vi "Generation Mode.vi"(8 "error in (no error)":errorcluster, 10 "Generation Mode":T1, 11 "PXIe5413 in":refnum<class "PXIe5413.lvclass">) -> (0 "error out":errorcluster, 3 "PXIe5413 out":refnum<class "PXIe5413.lvclass">)   [LabVIEW 2018, in "PXIe5413.lvlib" / "PXIe5413.lvclass"]
uses:
  PXIe5413.lvclass
  PPLs/Function Generator/Parent/Function Generator.lvlibp/Custom Controls/Generation Mode.ctl
  PPLs/Function Generator/Parent/Function Generator.lvlibp/Function Generator.lvclass
  C:/Projects/LabVIEW/PPLs/Function Generator/Parent/Function Generator.lvlibp/Function Generator.lvclass
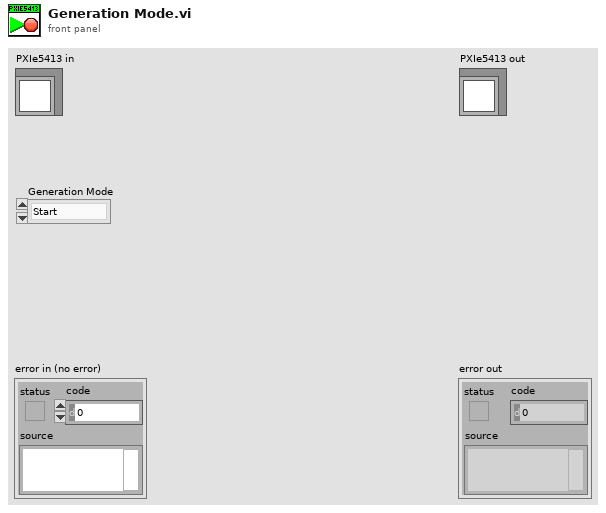
[diagram p1: front panel]
types:
  T1 = typedef "Function Generator.lvlibp/Function Generator.lvclass/Generation Mode.ctl" = enum16{"Start", "Stop"}
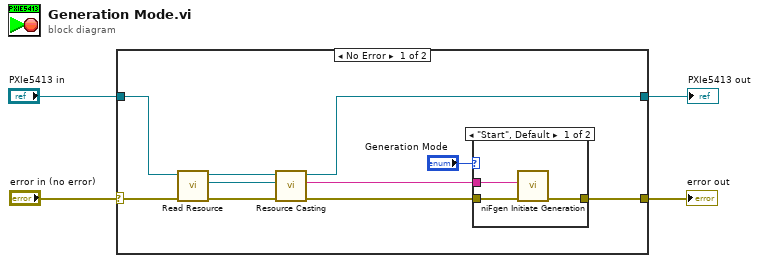
[diagram p0: block diagram]
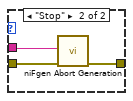
[diagram p2: hidden frame]
diagram:
  n1 = case shown="No Error" "error in (no error)" {
    selector: "error in (no error)" -> [w13 w22]
    tunnel: [w7 w22] -> w3
    tunnel: [w6 w21] -> w2
    tunnel: "PXIe5413 in" -> [w14 w21]
    frame No Error {
      n2 = call "Read Resource.vi"("error in (no error)"=w13, "Function Generator in"=w14) -> ("error out"=w12:errorcluster, "Resource"=w5:refnum<visa-resource-name>, "Function Generator out"=w11:refnum<class "PXIe5413.lvclass">)  [unwired: 7 in]
      n3 = call "Resource Casting.vi"("error in (no error)"=w12, "VISA Resource In"=w5, "PXIe5413 in"=w11) -> ("error out"=w10:errorcluster, "Casted Resource"=w8:string, "PXIe5413 out"=w6:refnum<class "PXIe5413.lvclass">)  [unwired: 6 in]
      n4 = case shown="\"Start\", Default" "Generation Mode" {
        tunnel: w10 -> [w17 w20]
        tunnel: w8 -> [w16 w18]
        tunnel: [w15 w19] -> w7
        frame "Start", Default {
          n5 = call <instrlib>:"niFgen Initiate Generation.vi"("error in (no error)"=w17, "Instrument Handle"=w16) -> ("error out"=w15:errorcluster)  [unwired: 8 in, 1 out]
        }
        frame "Stop" {
          n6 = call <instrlib>:"niFgen Abort Generation.vi"("error in (no error)"=w20, "Instrument Handle"=w18) -> ("error out"=w19:errorcluster)  [unwired: 8 in, 1 out]
        }
      }
    }
    frame Error {
    }
  }
  "error out" <- w3
  "PXIe5413 out" <- w2
